vi "Refresh SelectPoint Controls.vi"(8 "error in":errorcluster caption="错误输入（无错误）", 10 "Cmd":T1, 11 "Ctrls":T2) -> (0 "error out":errorcluster caption="错误输出")   [LabVIEW 2016]
uses:
  Ctrls/Select Point Operations.ctl
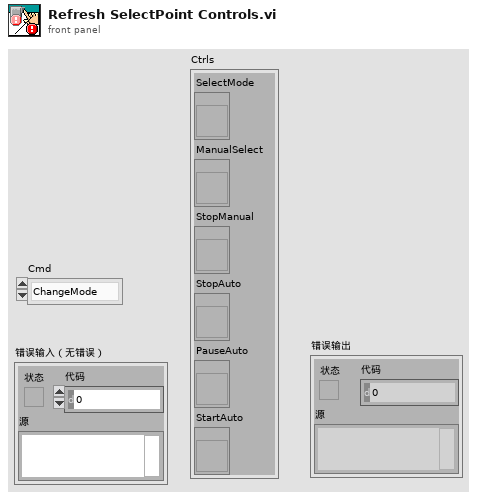
[diagram p1: front panel]
types:
  T1 = typedef "Select Point Operations.ctl" = enum16{"ChangeMode", "StartAuto", "PauseAuto", "StopAuto"}
  T2 = cluster{"SelectMode":refnum<vi>, "ManualSelect":refnum<vi>, "StopManual":refnum<vi>, "StopAuto":refnum<vi>, "PauseAuto":refnum<vi>, "StartAuto":refnum<vi>}
  T3 = enum8{"Enabled", "Disabled", "Disabled and Grayed Out"}
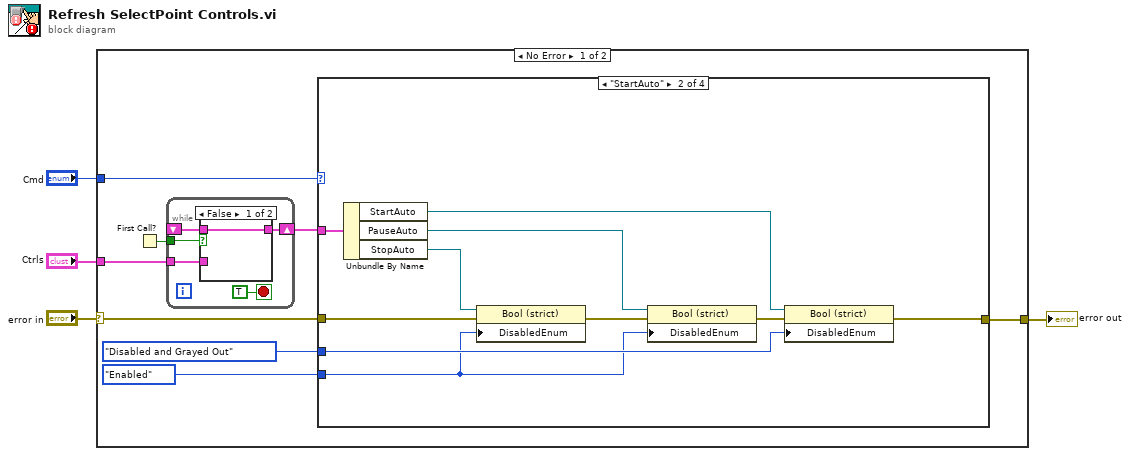
[diagram p0: block diagram]
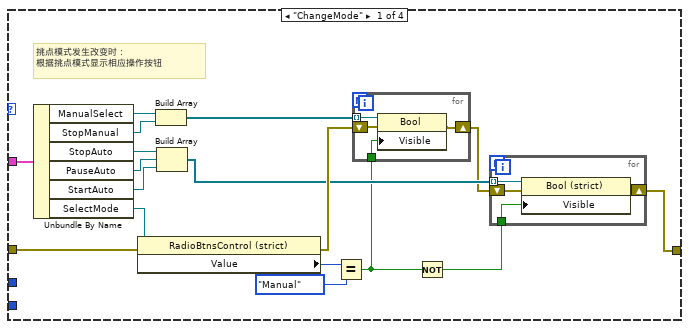
[diagram p3: hidden frame]
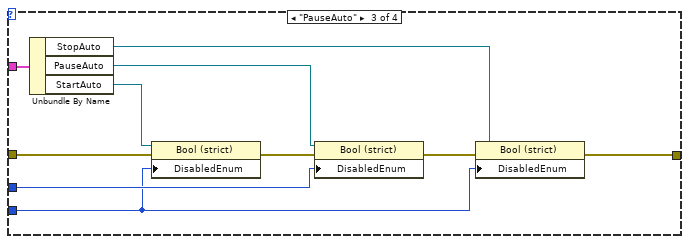
[diagram p4: hidden frame]
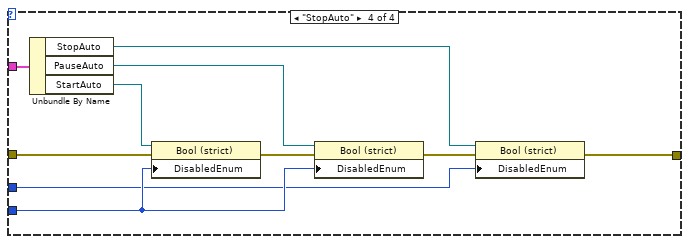
[diagram p5: hidden frame]
diagram:
  n1 = case shown="No Error" "error in" {
    selector: "error in" -> [w8 w75]
    tunnel: [w10 w75] -> w3
    tunnel: "Ctrls" -> [w6 _]
    tunnel: "Cmd" -> [w9 _]
    frame No Error {
      n2 = First Call?() -> (First Call?: T/F=w7:bool)
      n3 = while {
        shift-right: [w14] -> w5
        shift-left: _ -> [w15]
        tunnel: w7 -> [w16]
        tunnel: w6 -> [w13]
        stop <- TRUE stop-if-true
        n4 = case shown="False" w16 {
          tunnel: w15 -> [w18 _]
          tunnel: [w18 w19] -> w14
          tunnel: w13 -> [_ w19]
          frame False {
          }
          frame True {
          }
        }
      }
      n5 = case shown="\"StartAuto\"" w9 {
        tunnel: w8 -> [w34 w53 w63 w73]
        tunnel: w5 -> [w36 w54 w64 w74]
        tunnel: T3."Enabled" ("Disabled") -> [_ w45 w55 w66]
        tunnel: T3."Disabled and Grayed Out" ("Disabled") -> [_ w46 w56 w65]
        tunnel: [w21 w47 w57 w67] -> w10
        frame "ChangeMode" {
          # "挑点模式发生改变时：\n根据挑点模式显示相应操作按钮"
          n6 = Unbundle By Name(w36) -> ("ManualSelect"=w33:refnum<vi>, "StopManual"=w32:refnum<vi>, "StopAuto"=w31:refnum<vi>, "PauseAuto"=w30:refnum<vi>, "StartAuto"=w29:refnum<vi>, "SelectMode"=w35:refnum<vi>)
          n7 = property class="RadioBtnsControl (strict)"(reference=w35, error in=w34) -> (error out=w25:errorcluster, "Value"=w27:enum32{"Manual", "Auto"})  [unwired: 1 out]
          n8 = Build Array(w33, w32) -> (w28:refnum<vi>[])
          n9 = Build Array(w31, w30, w29) -> (w24:refnum<vi>[])
          n10 = Equal?(x=w27, y=enum32{"Manual", "Auto"}."Manual") -> (x = y?=w22:bool)
          n11 = for {
            tunnel: w28 -> [w44] mode=indexing
            tunnel: w22 -> [w43]
            shift-right: [w41] -> w23
            shift-left: w25 -> [w42]
            n12 = property class="Bool"(reference=w44, error in=w42, "Visible"=w43) -> (error out=w41:errorcluster)  [unwired: 1 out]
          }
          n13 = Not(x=w22) -> (.not. x?=w20:bool)
          n14 = for {
            tunnel: w24 -> [w40] mode=indexing
            tunnel: w20 -> [w39]
            shift-right: [w37] -> w21
            shift-left: w23 -> [w38]
            n15 = property class="Bool (strict)"(reference=w40, error in=w38, "Visible"=w39) -> (error out=w37:errorcluster)  [unwired: 1 out]
          }
        }
        frame "StartAuto" {
          n16 = Unbundle By Name(w54) -> ("StartAuto"=w48:refnum<vi>, "PauseAuto"=w50:refnum<vi>, "StopAuto"=w52:refnum<vi>)
          n17 = property class="Bool (strict)"(reference=w52, error in=w53, "DisabledEnum"=w45) -> (error out=w51:errorcluster)  [unwired: 1 out]
          n18 = property class="Bool (strict)"(reference=w50, error in=w51, "DisabledEnum"=w45) -> (error out=w49:errorcluster)  [unwired: 1 out]
          n19 = property class="Bool (strict)"(reference=w48, error in=w49, "DisabledEnum"=w46) -> (error out=w47:errorcluster)  [unwired: 1 out]
        }
        frame "PauseAuto" {
          n20 = Unbundle By Name(w64) -> ("StopAuto"=w58:refnum<vi>, "PauseAuto"=w60:refnum<vi>, "StartAuto"=w62:refnum<vi>)
          n21 = property class="Bool (strict)"(reference=w62, error in=w63, "DisabledEnum"=w55) -> (error out=w61:errorcluster)  [unwired: 1 out]
          n22 = property class="Bool (strict)"(reference=w60, error in=w61, "DisabledEnum"=w56) -> (error out=w59:errorcluster)  [unwired: 1 out]
          n23 = property class="Bool (strict)"(reference=w58, error in=w59, "DisabledEnum"=w55) -> (error out=w57:errorcluster)  [unwired: 1 out]
        }
        frame "StopAuto" {
          n24 = Unbundle By Name(w74) -> ("StopAuto"=w68:refnum<vi>, "PauseAuto"=w70:refnum<vi>, "StartAuto"=w72:refnum<vi>)
          n25 = property class="Bool (strict)"(reference=w72, error in=w73, "DisabledEnum"=w66) -> (error out=w71:errorcluster)  [unwired: 1 out]
          n26 = property class="Bool (strict)"(reference=w70, error in=w71, "DisabledEnum"=w66) -> (error out=w69:errorcluster)  [unwired: 1 out]
          n27 = property class="Bool (strict)"(reference=w68, error in=w69, "DisabledEnum"=w65) -> (error out=w67:errorcluster)  [unwired: 1 out]
        }
      }
    }
    frame Error {
    }
  }
  "error out" <- w3
